vi "Get Registry Update Event.vi"() -> (2 "Event Registration Refnum":refnum<event-registration>)   [LabVIEW 2020, in "Actor Framework.lvlib"]
doc: "This VI returns an Event registration refnum for an Actor Framework debugger to use to hear about changes to the available debug information of actors. Every time this event fires, new information from the database is available for the debugger to harvest and display. The event itself does not carry any information to avoid duplicating information in the Event queue."
uses:
  Actor Framework.lvlib
  tracing/Support/Registration Mode.ctl
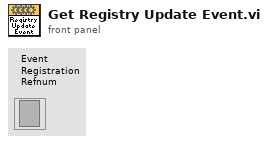
[diagram p1: front panel]
types:
  T1 = typedef "Actor Framework.lvlib/Registration Mode.ctl" = enum16{"Register Actor", "Get ID", "Get Enqueuer", "Deregister Actor", "Get Update Event", "Get All Actors", "Set Actor Core Name"}
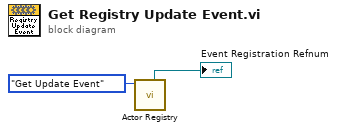
[diagram p0: block diagram]
diagram:
  n1 = call "Actor Registry.vi"("Action"=Registration_Mode."Get Update Event") -> ("Event Registration Refnum"=→"Event Registration Refnum":refnum<event-registration>)  [unwired: 6 in, 4 out]
